vi "CRYSet Stimulus Editor Front Panel.vi"(11 "Vi Ref":refnum<vi>) -> ()   [LabVIEW 2013]
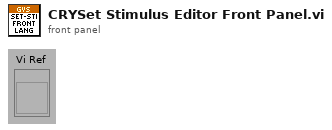
[diagram p1: front panel]
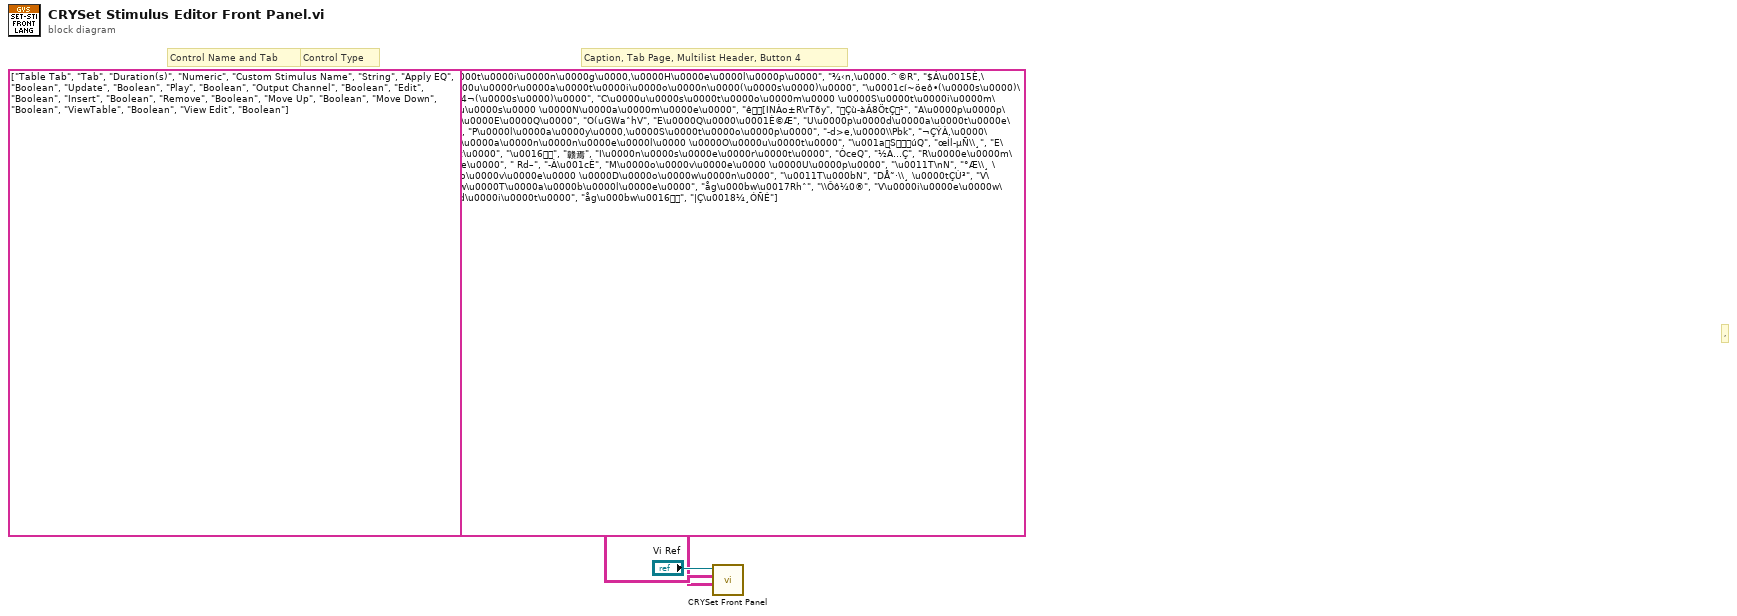
[diagram p0: block diagram]
diagram:
  # ","
  # "Caption, Tab Page, Multilist Header, Button 4"
  # "Control Type"
  # "Control Name and Tab"
  n1 = call "CRYSet Front Panel.vi"("Caption(Boolean Text)"=string[][] [["S\u0000e\u0000t\u0000t\u0000i\u0000n\u0000g\u0000,\u0000H\u0000e\u0000l\u0000p\u0000", "¾‹n,\u0000.^©R", "$Á\u0015È,\u0000Ä³ÀÆÐ¹"], ["D\u0000u\u0000r\u0000a\u0000t\u0000i\u0000o\u0000n\u0000(\u0000s\u0000)\u0000", "\u0001cí~öeô•(\u0000s\u0000)\u0000", "ÀÉÁÜÂ\u0004¬(\u0000s\u0000)\u0000"], ["C\u0000u\u0000s\u0000t\u0000o\u0000m\u0000 \u0000S\u0000t\u0000i\u0000m\u0000u\u0000l\u0000u\u0000s\u0000 \u0000N\u0000a\u0000m\u0000e\u0000", "ê[INÀo±R\rTðy", "Çù­àÂ8ÖtÇ¹"], ["A\u0000p\u0000p\u0000l\u0000y\u0000 \u0000E\u0000Q\u0000", "O(uGWaˆhV", "E\u0000Q\u0000\u0001È©Æ"], ["U\u0000p\u0000d\u0000a\u0000t\u0000e\u0000", "ôf°e", "1¬àÂ"], ["P\u0000l\u0000a\u0000y\u0000,\u0000S\u0000t\u0000o\u0000p\u0000", "­d>e,\u0000\\Pbk", "¬ÇÝÀ,\u0000\u0015ÈÀÉ"], ["C\u0000h\u0000a\u0000n\u0000n\u0000e\u0000l\u0000 \u0000O\u0000u\u0000t\u0000", "\u001aSúQ", "œÍl­µÑ\\¸"], ["E\u0000d\u0000i\u0000t\u0000", "\u0016", "赣焉"], ["I\u0000n\u0000s\u0000e\u0000r\u0000t\u0000", "ÒceQ", "½À…Ç"], ["R\u0000e\u0000m\u0000o\u0000v\u0000e\u0000", " Rd–", "­À\u001cÈ"], ["M\u0000o\u0000v\u0000e\u0000 \u0000U\u0000p\u0000", "\u0011T\nN", "°Æ\\¸ \u0000tÇÙ³"], ["M\u0000o\u0000v\u0000e\u0000 \u0000D\u0000o\u0000w\u0000n\u0000", "\u0011T\u000bN", "DÅ˜·\\¸ \u0000tÇÙ³"], ["V\u0000i\u0000e\u0000w\u0000T\u0000a\u0000b\u0000l\u0000e\u0000", "åg\u000bw\u0017Rhˆ", "\\Ôô¼0®"], ["V\u0000i\u0000e\u0000w\u0000 \u0000E\u0000d\u0000i\u0000t\u0000", "åg\u000bw\u0016", "|Ç\u0018¼¸ÓÑÉ"]], "Control ID and Type(Label Name, Type)"=string[][] [["Table Tab", "Tab"], ["Duration(s)", "Numeric"], ["Custom Stimulus Name", "String"], ["Apply EQ", "Boolean"], ["Update", "Boolean"], ["Play", "Boolean"], ["Output Channel", "Boolean"], ["Edit", "Boolean"], ["Insert", "Boolean"], ["Remove", "Boolean"], ["Move Up", "Boolean"], ["Move Down", "Boolean"], ["ViewTable", "Boolean"], ["View Edit", "Boolean"]], "Vi Ref"="Vi Ref") -> ()  [unwired: 9 in]
